vi "PictureControl_GetTextRect.vi"(0 "alignment(left, top)":T2, 1 "desired font(Application)":T4(ring)=enum."Application Font", 2 "origin(0,0)":cluster{"horizontal":i16, "vertical":i16}, 3 "text":string, 4 "text orientation":T1(ring), 5 "[user-specified font]":T5) -> (7 "rect":T3)   [LabVIEW 2020]
doc: "Returns a cluster that contains the left, top, right, and bottom dimensions, in pixels, of a string."
panel:
  out "NumberOfSavedSizes":i32
  in  "used only for\ndatatype":T3
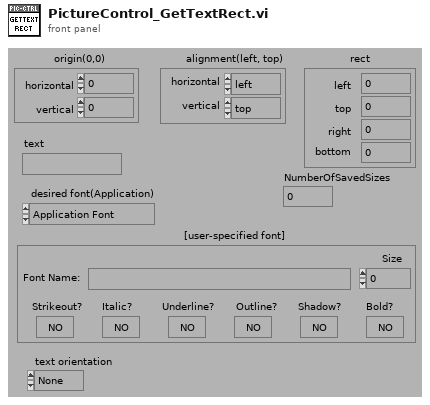
[diagram p1: front panel]
types:
  T1 = enum16{"None", "Stacked", "Clockwise", "Counterclockwise"}
  T2 = cluster{"horizontal":enum16{"left", "center", "right"}, "vertical":enum16{"top", "center", "bottom"}}
  T3 = cluster{"left":i16, "top":i16, "right":i16, "bottom":i16}
  T4 = enum16{"User-specified Font", "Application Font", "System Font", "Dialog Font"}
  T5 = cluster{"Font Name:":string, "Size":i16, "Strikeout?":bool, "Italic?":bool, "Underline?":bool, "Outline?":bool, "Shadow?":bool, "Bold?":bool}
  T6 = cluster{"text":string, i32, "[user-specified font]":cluster{"Font Name:":string, "Size":i16, "Strikeout?":bool, "Italic?":bool, "Underline?":bool, "Outline?":bool, "Shadow?":bool, "Bold?":bool}, i32}
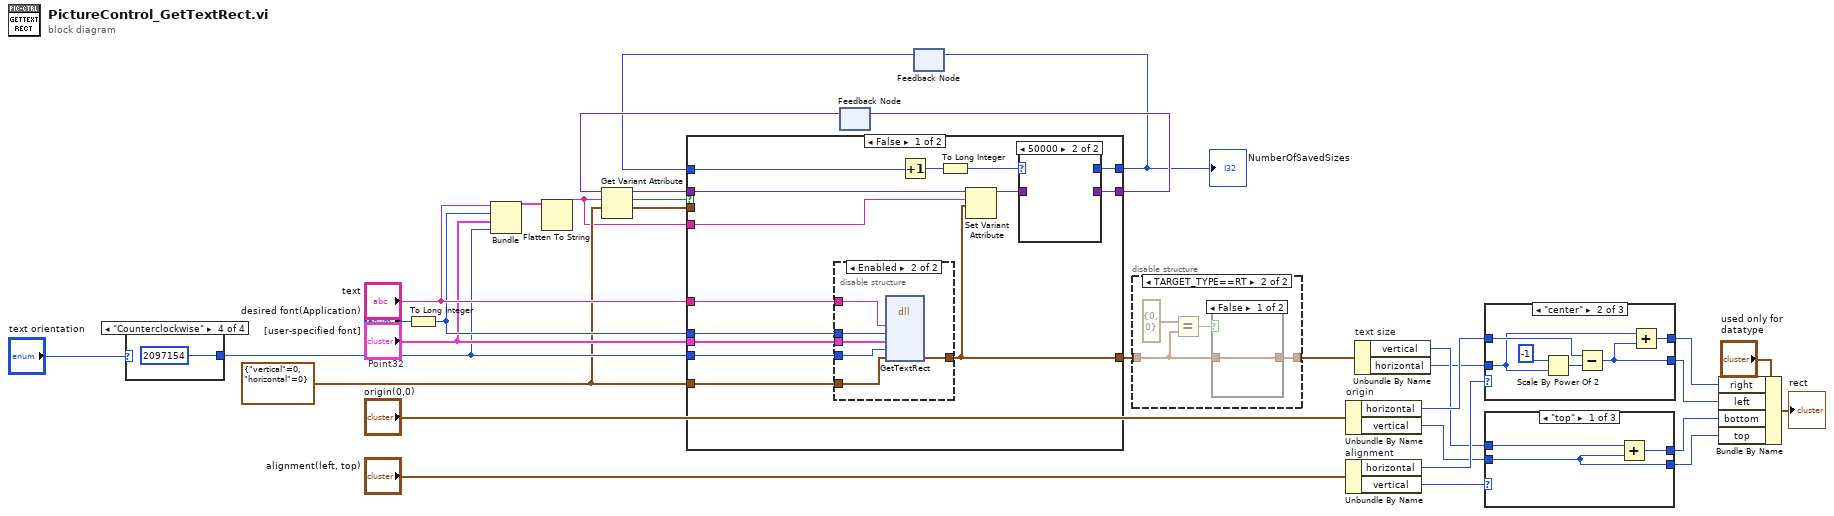
[diagram p0: block diagram]
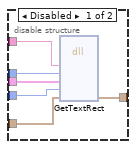
[diagram p3: hidden frame]
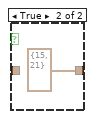
[diagram p6: hidden frame]
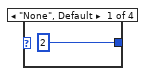
[diagram p7: hidden frame]
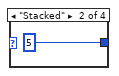
[diagram p8: hidden frame]
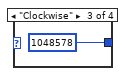
[diagram p9: hidden frame]
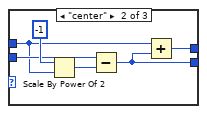
[diagram p10: hidden frame]
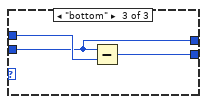
[diagram p11: hidden frame]
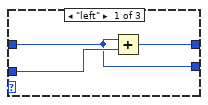
[diagram p12: hidden frame]
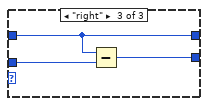
[diagram p13: hidden frame]
diagram:
  w8 = cluster{"vertical":i32, "horizontal":i32} {"vertical"=0, "horizontal"=0}
  # "Point32"
  n1 = case shown="\"Counterclockwise\"" "text orientation" {
    tunnel: [2 5 1048578 2097154] -> w11
    frame "None", Default {
    }
    frame "Stacked" {
    }
    frame "Clockwise" {
    }
    frame "Counterclockwise" {
    }
  }
  n2 = To Long Integer(number="desired font(Application)") -> (32bit integer=w13:i32)
  n3 = Bundle("text"="text", w13, "[user-specified font]"="[user-specified font]", w11) -> (w10:T6)  [unwired: 1 in]
  n4 = Flatten To String(anything=w10) -> (data string=w4:string)  [unwired: 3 in, 2 out]
  n5 = feedback #1() -> (w9:variant)  [unwired: 1 in]
  n6 = Get Variant Attribute(Variant=w9, name=w4, default value (empty Variant)=w8) -> (duplicate Variant=w6:variant, found=w7:bool, value=w5:cluster{"vertical":i32, "horizontal":i32})  [unwired: 1 in, 1 out]
  n7 = feedback #2() -> (w1:i32)  [unwired: 1 in]
  n8 = case shown="False" w7 {
    tunnel: [w43 w66] -> w16
    tunnel: "text" -> [w50 _]
    tunnel: w13 -> [w49 _]
    tunnel: "[user-specified font]" -> [w48 _]
    tunnel: w11 -> [w47 _]
    tunnel: w8 -> [w46 _]
    tunnel: w6 -> [w45 w67]
    tunnel: [w37 w67] -> w3
    tunnel: w5 -> [_ w66]
    tunnel: w4 -> [w44 _]
    tunnel: [w38 w65] -> w2
    tunnel: w1 -> [w41 w65]
    frame False {
      n9 = disable-structure shown="Enabled" {
        disable-tunnel: w50 -> [w58 w64]
        disable-tunnel: w49 -> [w57 w63]
        disable-tunnel: w48 -> [w56 w62]
        disable-tunnel: w46 -> [w55 w61]
        disable-tunnel: w47 -> [w54 w60]
        disable-tunnel: [w53 w59] -> w43
        frame Disabled {
          n10 = dll-call lib="LabVIEW" fn="GetTextRect"("string"=w58, "desiredFont"=w57, "userSpecifiedFont"=w56, "mode"=w54, "extents"=w55) -> ("extents"=w53:cluster{"vertical":i32, "horizontal":i32})  [unwired: 8 in, 2 out]
        }
        frame Enabled {
          n11 = dll-call lib="LabVIEW" fn="GetTextRect"("string"=w64, "desiredFont"=w63, "userSpecifiedFont"=w62, "mode"=w60, "extents"=w61) -> ("extents"=w59:cluster{"vertical":i32, "horizontal":i32})  [unwired: 8 in, 2 out]
        }
      }
      n12 = Increment(x=w41) -> (x+1=w42:i32)
      n13 = To Long Integer(number=w42) -> (32bit integer=w40:i32)
      n14 = Set Variant Attribute(Variant=w45, name=w44, value=w43) -> (Variant out=w39:variant)  [unwired: 1 in, 2 out]
      n15 = case shown="50000" w40 {
        selector: w40 -> [w52 _]
        tunnel: w39 -> [w51 _]
        tunnel: [w52 _] -> w38
        tunnel: [w51 _] -> w37
        frame 0, Default {
        }
        frame 50000 {
        }
      }
    }
    frame True {
    }
  }
  "NumberOfSavedSizes" <- w2
  n16 = feedback-in #1(w3) -> ()
  n17 = feedback-in #2(w2) -> ()
  n18 = disable-structure shown="TARGET_TYPE==RT" {
    disable-tunnel: [w68 w72] -> w15
    disable-tunnel: w16 -> [w68 w69]
    frame condition #0 (active) {
    }
    frame condition #1 {
      n19 = Equal?(x=cluster{"vertical":i32, "horizontal":i32} {"vertical"=0, "horizontal"=0} ("output param"), y=w69) -> (x = y?=w71:bool)
      n20 = case shown="False" w71 {
        tunnel: [w73 cluster{"vertical":i32, "horizontal":i32} {"vertical"=15, "horizontal"=21} ("output param")] -> w72
        tunnel: w69 -> [w73 _]
        frame False {
        }
        frame True {
        }
      }
    }
  }
  n21 = Unbundle By Name "origin"("origin(0,0)") -> ("horizontal"=w27:i16, "vertical"=w23:i16)
  n22 = Unbundle By Name "alignment"("alignment(left, top)") -> ("horizontal"=w28:enum16{"left", "center", "right"}, "vertical"=w24:enum16{"top", "center", "bottom"})
  n23 = Unbundle By Name "text size"(w15) -> ("vertical"=w19:i32, "horizontal"=w18:i32)
  n24 = case shown="\"center\"" w28 {
    tunnel: w18 -> [w76 w78 w86]
    tunnel: w27 -> [w75 w79 w84]
    tunnel: [w75 w81 w85] -> w26
    tunnel: [w77 w80 w84] -> w25
    frame "left" {
      n25 = Add(x=w75, y=w76) -> (x+y=w77:i32)
    }
    frame "center" {
      n26 = Scale By Power Of 2(n=-1, x=w78) -> (x*2^n=w82:i32)
      n27 = Subtract(x=w79, y=w82) -> (x-y=w81:i32)
      n28 = Add(x=w78, y=w81) -> (x+y=w80:i32)
    }
    frame "right" {
      n29 = Subtract(x=w84, y=w86) -> (x-y=w85:i32)
    }
  }
  n30 = case shown="\"top\"" w24 {
    tunnel: w19 -> [w88 w90 w98]
    tunnel: w23 -> [w87 w91 w96]
    tunnel: [w87 w93 w97] -> w22
    tunnel: [w89 w92 w96] -> w21
    frame "top" {
      n31 = Add(x=w88, y=w87) -> (x+y=w89:i32)
    }
    frame "center" {
      n32 = Scale By Power Of 2(n=-1, x=w90) -> (x*2^n=w94:i32)
      n33 = Subtract(x=w91, y=w94) -> (x-y=w93:i32)
      n34 = Add(x=w90, y=w93) -> (x+y=w92:i32)
    }
    frame "bottom" {
      n35 = Subtract(x=w96, y=w98) -> (x-y=w97:i32)
    }
  }
  n36 = Bundle By Name(cluster="used only for\ndatatype", "right"=w25, "left"=w26, "bottom"=w21, "top"=w22) -> (→"rect":T3)
